vi "Save Errors Info next to LV Project.vi"(10 "Errors Info":string[][](array[string]), 11 "Project Path":path) -> ()   [LabVIEW 2020, in "ConstantErrorsMaker.lvlib"]
uses:
  ConstantErrorsMaker.lvlib
  <vilib>/Utility/file.llb/Write Delimited Spreadsheet (string).vi
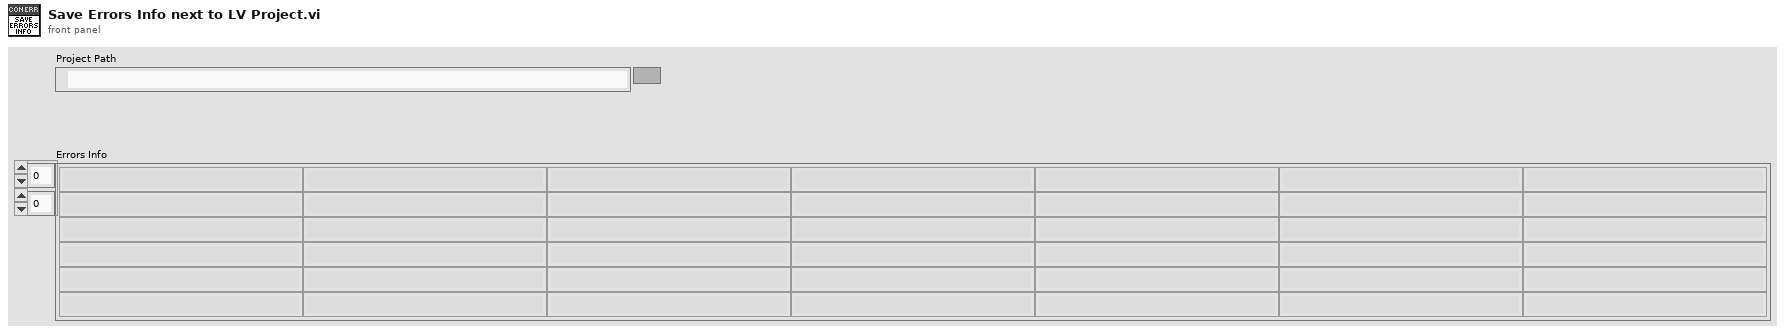
[diagram p1: front panel]
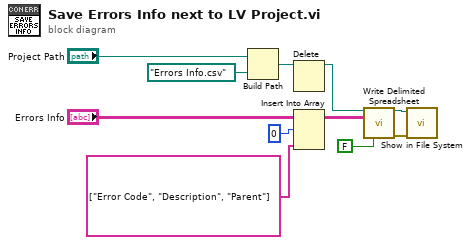
[diagram p0: block diagram]
diagram:
  n1 = Build Path(base path="Project Path", name or relative path=path "Errors Info.csv") -> (appended path=w6:path)
  n2 = Delete(path (use dialog)=w6) -> (deleted path=w7:path)  [unwired: 4 in, 2 out]
  n3 = Insert Into Array(array="Errors Info", index (row)=0, new element=string[] ["Error Code", "Description", "Parent"]) -> (w9:string[][])  [unwired: 1 in]
  n4 = call-poly <vilib>:"Write Delimited Spreadsheet.vi"("file path (dialog if empty)"=w7, "2D data"=w9, "transpose? (no:F)"=FALSE) -> ("new file path (Not A Path if cancelled)"=w4:path, "error out"=w11:errorcluster)  [unwired: 11 in]
  n5 = call <vilib>:"Show in File System.vi"("error in (no error)"=w11, "file or directory path"=w4) -> ()  [unwired: 9 in, 1 out]
